vi "Sub3.vi"() -> ()   [LabVIEW 2018]
panel:
  out "Sun Lon":dbl
  out "Sun Lat":dbl
  in  "Path to PNG file":path
  out "XY Graph":cluster{dbl[], dbl[]}[](graph)
  out "error out":errorcluster
  in  "error in (no error)":errorcluster
  in  "URL":string
  in  "Stop":bool
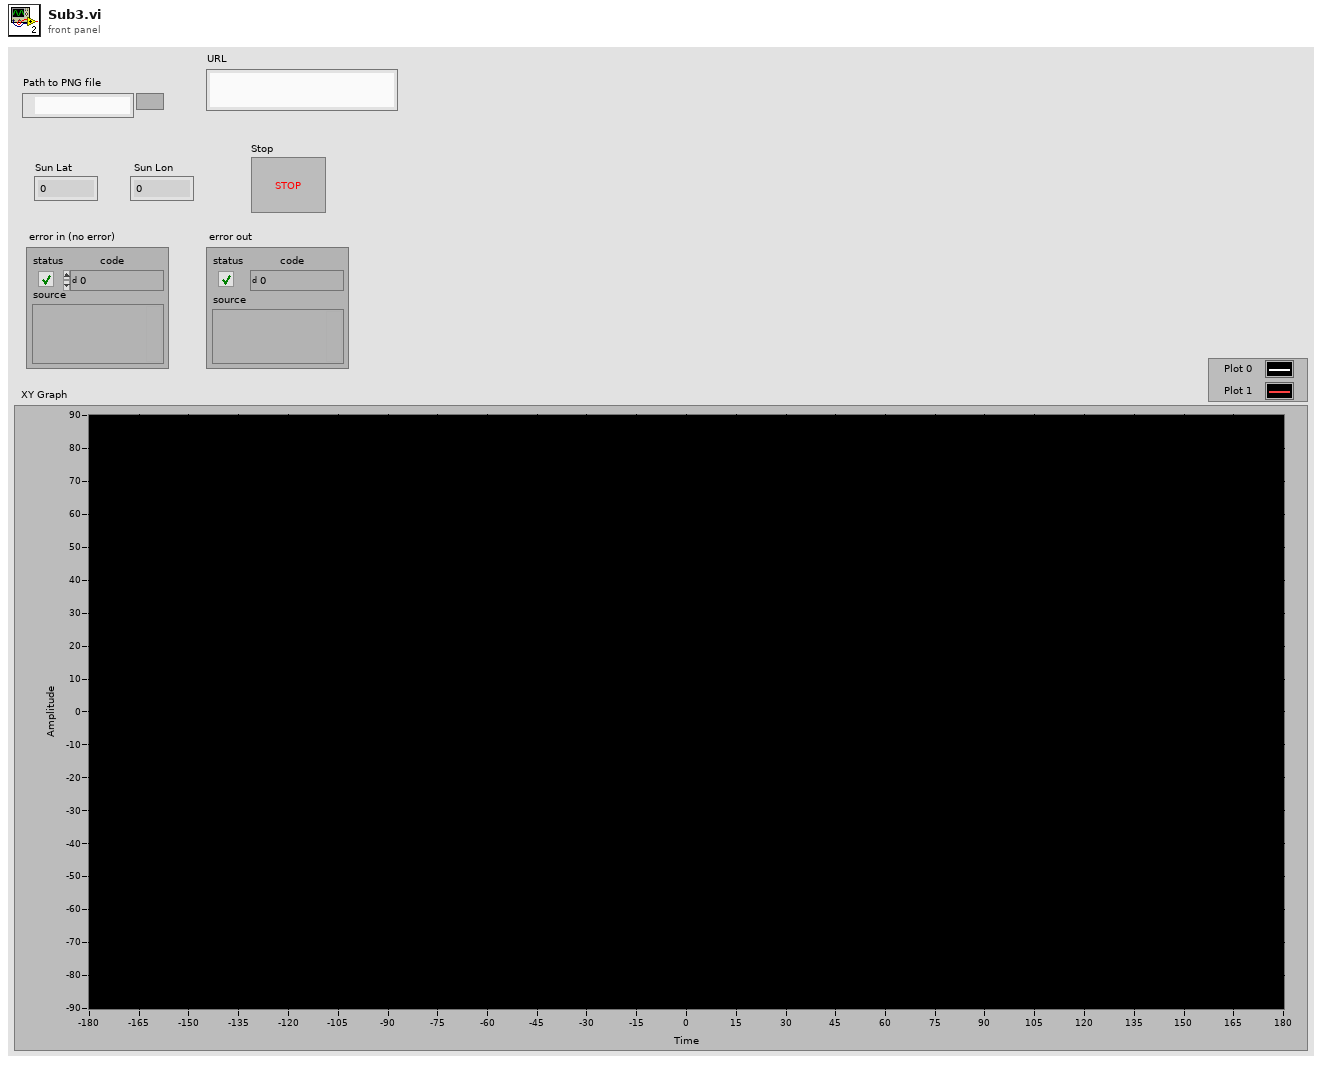
[diagram p1: front panel]
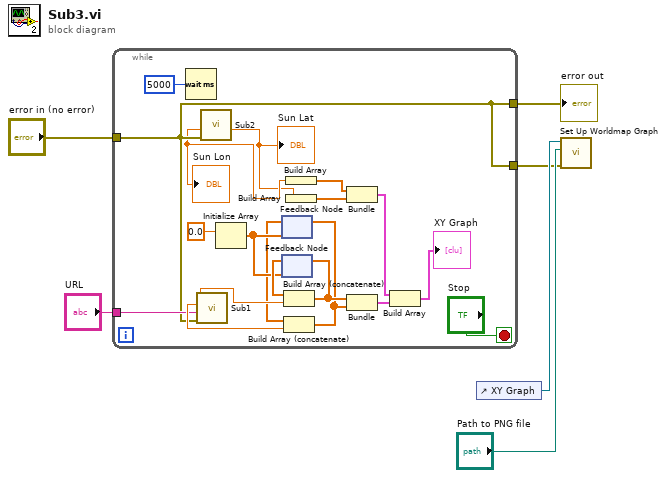
[diagram p0: block diagram]
diagram:
  n1 = while {
    tunnel: "URL" -> [w15]
    tunnel: [w9] -> w5
    tunnel: "error in (no error)" -> [w9]
    tunnel: [w9] -> w1
    stop <- "Stop" stop-if-true
    n2 = Wait (ms)(milliseconds to wait=u32 5000) -> ()  [unwired: 1 out]
    n3 = call "Sub1.vi"("error in (no error)"=w9, "URL"=w15) -> ("ISS Lat"=w19:dbl, "ISS Lon"=w20:dbl)  [unwired: 7 in, 1 out]
    n4 = call "Sub2.vi"("error in (no error)"=w9) -> ("Sun Lat"=w7:dbl, "Sun Lon"=w8:dbl)  [unwired: 8 in, 1 out]
    "Sun Lat" <- w7
    "Sun Lon" <- w8
    n5 = Initialize Array(0.0 ("element")) -> (w21:dbl[])  [unwired: 1 in]
    n6 = feedback #1(w21) -> (w18:dbl[])
    n7 = feedback #2(w21) -> (w23:dbl[])
    n8 = Build Array (concatenate)(w23, w20) -> (w17:dbl[])
    n9 = feedback-in #2(w17) -> ()
    n10 = Build Array (concatenate)(w18, w19) -> (w16:dbl[])
    n11 = feedback-in #1(w16) -> ()
    n12 = Build Array(w8) -> (w14:dbl[])
    n13 = Build Array(w7) -> (w13:dbl[])
    n14 = Bundle(w14, w13) -> (w12:cluster{dbl[], dbl[]})  [unwired: 1 in]
    n15 = Bundle(w17, w16) -> (w11:cluster{dbl[], dbl[]})  [unwired: 1 in]
    n16 = Build Array(w12, w11) -> (→"XY Graph":cluster{dbl[], dbl[]}[])
  }
  "error out" <- w5
  n17 = control-ref of="XY Graph"() -> (w3:refnum<vi>)
  n18 = call "Set Up Worldmap Graph.vi"("error in (no error)"=w1, "Path to PNG file"="Path to PNG file", "XYGraph Refnum"=w3) -> ()  [unwired: 8 in, 1 out]
